vi "Read Motor Param.vi"(8 "error in (no error)":errorcluster, 10 "Address":u16=4102 format="%.0x", 11 "FujiMotor in":refnum<class "FujiMotor.lvclass">) -> (0 "error out":errorcluster, 3 "FujiMotor out":refnum<class "FujiMotor.lvclass">)   [LabVIEW 2014, in "ALPHA5 RS485.lvlib" / "FujiMotor.lvclass"]
uses:
  FujiMotor.lvclass
  FujiMotor.lvclass/FujiMotor.ctl
  ALPHA5 RS485.lvlib
panel:
  out "Value":i32
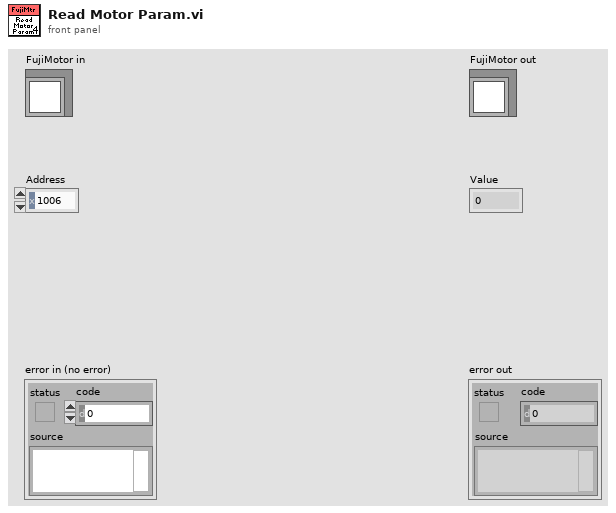
[diagram p1: front panel]
types:
  T1 = typedef "ALPHA5 RS485.lvlib/Port Selection Info.ctl" = cluster{"Port Name":refnum<visa-resource-name>, "Amplifier Num":u8, "Baud Rate":u32, "Char Formation":enum16{"0", "1", "2", "3", "4", "5"}}
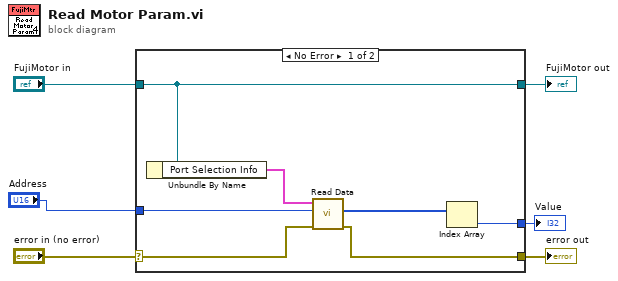
[diagram p0: block diagram]
diagram:
  n1 = case shown="No Error" "error in (no error)" {
    selector: "error in (no error)" -> [w11 w14]
    tunnel: [w10 w14] -> w5
    tunnel: [w13 w15] -> w3
    tunnel: "FujiMotor in" -> [w13 w15]
    tunnel: [w8 _] -> w2
    tunnel: "Address" -> [w7 _]
    frame No Error {
      n2 = Unbundle By Name(w13) -> ("Port Selection Info"=w12:T1)
      n3 = call "Read Data.vi"("error in (no error)"=w11, "Address"=w7, "Port Selection Info In"=w12) -> ("error out"=w10:errorcluster, "Data"=w9:u32[])  [unwired: 5 in, 2 out]
      n4 = Index Array(array=w9) -> (element=w8:u32)  [unwired: 1 in]
    }
    frame Error {
    }
  }
  "error out" <- w5
  "FujiMotor out" <- w3
  "Value" <- w2
